vi "Get Connection.vi"(8 "error in (no error)":errorcluster) -> (0 "error out":errorcluster, 3 "connection":T1)   [LabVIEW 2021, in "AudioGenManageConnectionProcess.lvlib"]
uses:
  AudioGenManageConnectionProcess.lvlib
  <vilib>/NI/STM/TCP/TCP Connection Info.ctl
  <vilib>/NI/STM/SubVIs/MetaDataElement.ctl
  <vilib>/addons/PointValueMap/subVIs/Point_Read_variant.vi
  <vilib>/addons/PointValueMap/PointValueMap.lvlib
  <vilib>/NI/STM/NI STM.lvlib
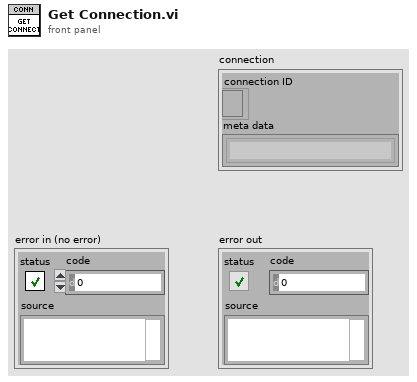
[diagram p1: front panel]
types:
  T1 = typedef "NI STM.lvlib/TCP Connection Info.ctl" = cluster{"connection ID":refnum<k5>, "meta data":T2[]}
  T2 = typedef "NI STM.lvlib/MetaDataElement.ctl" = string
  T3 = typedef "PointValueMap.lvlib/PointMap.ctl" = refnum<data-value>
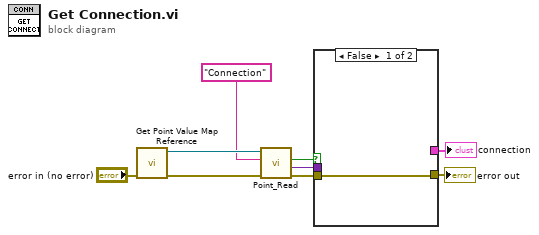
[diagram p0: block diagram]
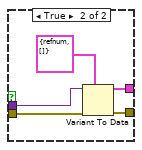
[diagram p2: hidden frame]
diagram:
  n1 = call "Get Point Value Map Reference.vi"("error in (no error)"="error in (no error)") -> ("error out"=w7:errorcluster, "Map Out"=w8:T3)  [unwired: 9 in]
  n2 = call-poly <vilib>:"Point_Read.vi"("Error In"=w7, "Tag"="Connection", "Map"=w8) -> ("Error Out"=w5:errorcluster, "Value"=w3:variant, "Found?"=w1:bool)  [unwired: 3 in, 3 out]
  n3 = case shown="False" w1 {
    tunnel: w5 -> [w10 w15]
    tunnel: [w10 w14] -> w4
    tunnel: w3 -> [_ w13]
    tunnel: [_ w11] -> w2
    frame False {
    }
    frame True {
      n4 = Variant To Data(error in=w15, type=T1 {"connection ID"=refnum, "meta data"=[]} ("connection"), Variant=w13) -> (data=w11:T1, error out=w14:errorcluster)
    }
  }
  "connection" <- w2
  "error out" <- w4
